vi "Defer Panel Update.vi"(8 "error in (no error)":errorcluster, 10 "Defer Panel Updates":bool, 11 "UI_Actor in":refnum<class "UI_Actor.lvclass">) -> (0 "error out":errorcluster, 3 "UI_Actor out":refnum<class "UI_Actor.lvclass">)   [LabVIEW 2020, in "UI_Actor.lvlib" / "UI_Actor.lvclass"]
uses:
  UI_Actor.lvclass
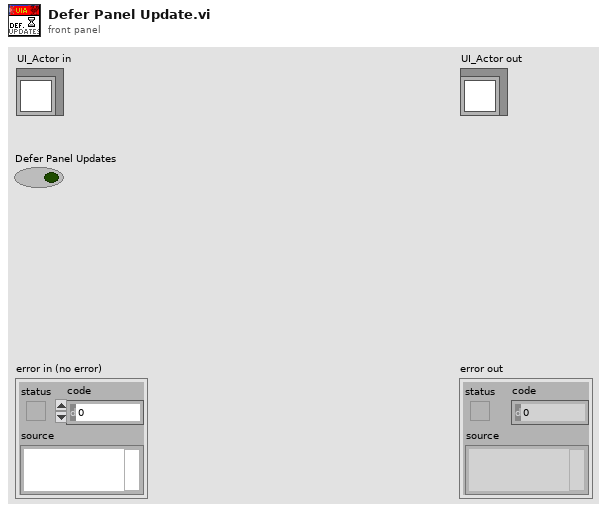
[diagram p1: front panel]
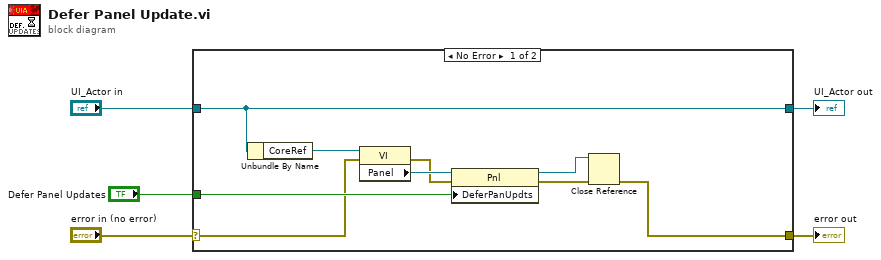
[diagram p0: block diagram]
diagram:
  n1 = case shown="No Error" "error in (no error)" {
    selector: "error in (no error)" -> [w10 w16]
    tunnel: [w6 w16] -> w4
    tunnel: [w14 w15] -> w2
    tunnel: "UI_Actor in" -> [w14 w15]
    tunnel: "Defer Panel Updates" -> [w11 _]
    frame No Error {
      n2 = Unbundle By Name(w14) -> ("CoreRef"=w13:refnum<vi>)
      n3 = property class="VI"(reference=w13, error in=w10) -> (error out=w9:errorcluster, "Panel"=w12:refnum<vi>)  [unwired: 1 out]
      n4 = property class="Pnl"(reference=w12, error in=w9, "DeferPanUpdts"=w11) -> (reference out=w8:refnum<vi>, error out=w7:errorcluster)
      n5 = Close Reference(reference=w8, error in (no error)=w7) -> (error out=w6:errorcluster)
    }
    frame Error {
    }
  }
  "error out" <- w4
  "UI_Actor out" <- w2
